vi "System.vi"() -> ()   [LabVIEW 2015]
panel:
  in  "權限管理":bool
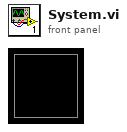
[diagram p1: front panel]
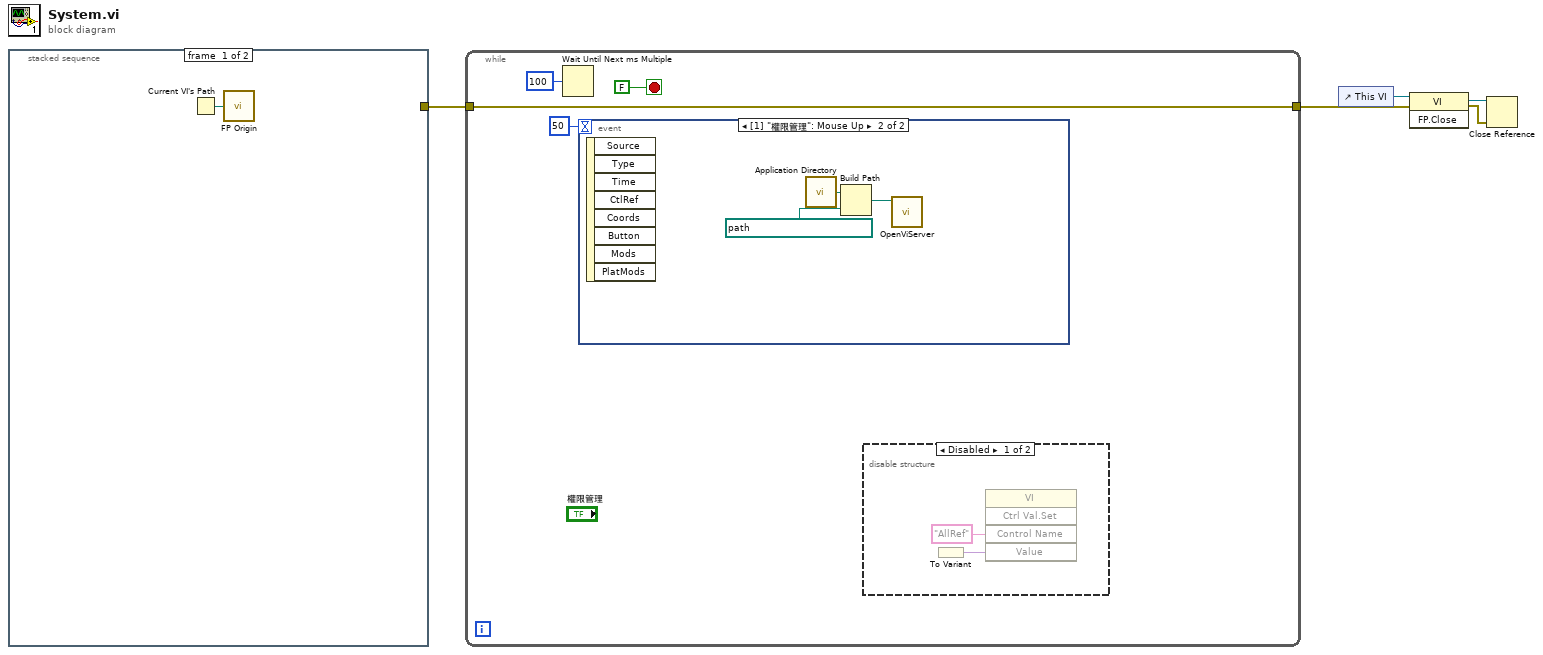
[diagram p0: block diagram]
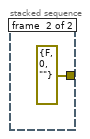
[diagram p2: hidden frame]
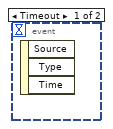
[diagram p4: hidden frame]
diagram:
  n1 = stacked-sequence {
    tunnel: [_ errorcluster {"status"=FALSE, "code"=0, "source"=""} ("error out")] -> w1
    frame #0 {
      n2 = Current VI's Path() -> (path=w6:path)
      n3 = call "FP Origin.vi"("vi path"=w6) -> ()  [unwired: 1 out]
    }
    frame #1 {
    }
  }
  n4 = while {
    tunnel: w1 -> [w9]
    tunnel: [w9] -> w5
    stop <- FALSE stop-if-true
    n5 = Wait Until Next ms Multiple(millisecond multiple=u32 100) -> ()  [unwired: 1 out]
    n6 = event shown="[1] \"權限管理\": Mouse Up" {
      selector: _ -> [_ _]
      dyn-events: _ -> [_ _]
      timeout: 50 -> [_ _]
      event Timeout {
        n7 = event-data() -> ()  [unwired: 1 in, 3 out]
      }
      event "權限管理": Mouse Up {
        n8 = event-data() -> ()  [unwired: 1 in, 8 out]
        n9 = call <vilib>:"Application Directory.vi"() -> ("Application Directory"=w17:path)
        n10 = Build Path(base path=w17, name or relative path=path "0.Main/檔案_權限密碼.vi" ("vi path")) -> (appended path=w15:path)
        n11 = call "OpenViServer.vi"("vi path"=w15) -> ()  [unwired: 9 in, 2 out]
      }
    }
    n12 = disable-structure shown="Disabled" {
      frame Disabled {
        n13 = To Variant() -> (Variant=w13:variant)  [unwired: 1 in]
        n14 = invoke class="VI" method="Ctrl Val.Set"("Control Name"="AllRef", "Value"=w13) -> (error in=w12:errorcluster)  [unwired: 2 in, 5 out]
      }
      frame Enabled {
      }
    }
  }
  n15 = control-ref of="This VI"() -> (w4:refnum<vi>)
  n16 = invoke class="VI" method="FP.Close"(reference=w4, error in=w5) -> (reference out=w3:refnum<vi>, error out=w2:errorcluster)  [unwired: 1 in, 1 out]
  n17 = Close Reference(reference=w3, error in (no error)=w2) -> ()  [unwired: 1 out]
